vi "Process.vi"(8 "error in":errorcluster, 11 "Qbus in":refnum<class "Qbus.lvclass">) -> (0 "error out":errorcluster)   [LabVIEW 2021, in "TemplateProcess.lvlib"]
uses:
  TemplateProcess.lvlib
  <vilib>/addons/Qbus/Qbus.lvclass
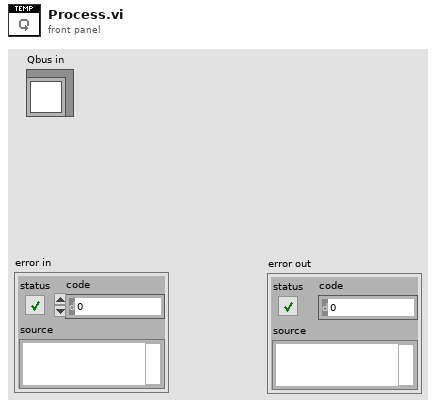
[diagram p1: front panel]
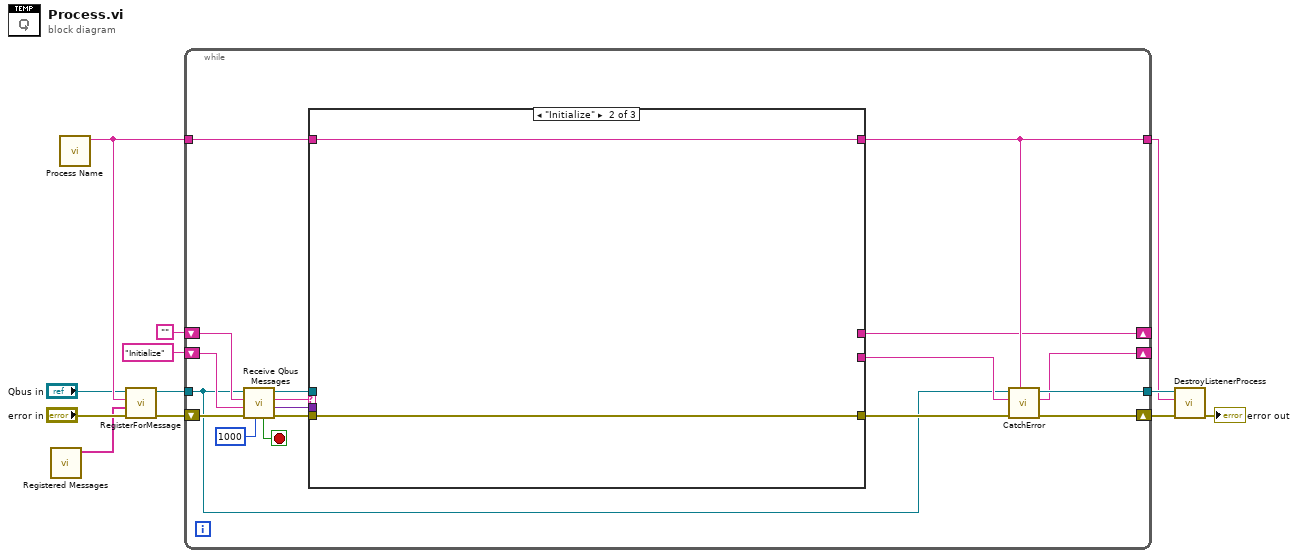
[diagram p0: block diagram]
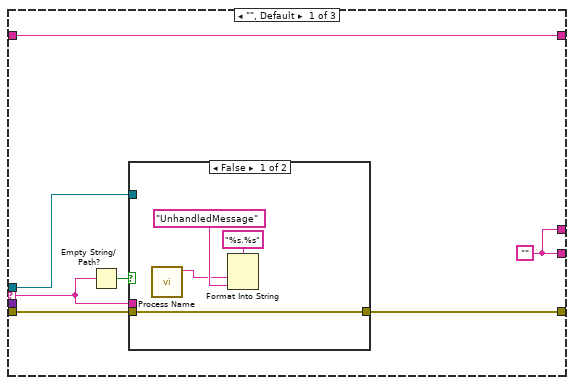
[diagram p2: hidden frame]
diagram:
  n1 = call "Registered Messages.vi"() -> ("registered messages"=w5:string[])  [unwired: 11 in]
  n2 = call "Process Name.vi"() -> ("process name"=w8:string)  [unwired: 11 in]
  n3 = call <vilib>:"RegisterForMessage.vi"("error in (no error)"="error in", "message names"=w5, "process name"=w8, "Qbus in"="Qbus in") -> ("error in (no error)"=w11:errorcluster, "Qbus out"=w12:refnum<class "Qbus.lvclass">)  [unwired: 6 in]
  n4 = while {
    shift-right: [w16] -> _
    shift-left: "" -> [w29]
    tunnel: w12 -> [w14]
    tunnel: w8 -> [w13]
    tunnel: [w23] -> w3
    tunnel: [w18] -> w1
    shift-right: [w22] -> _
    shift-left: "Initialize" -> [w25]
    shift-right: [w24] -> w4
    shift-left: w11 -> [w21]
    stop <- w30 stop-if-true
    n5 = call "Receive Qbus Messages.vi"("timeout(ms)"=1000 ("milliseconds to wait"), "error in (no error)"=w21, "priority action"=w25, "default action"=w29, "Qbus in"=w14) -> ("error out"=w28:errorcluster, "message value"=w26:variant, "action"=w20:string, "Qbus out"=w27:refnum<class "Qbus.lvclass">, "exit"=w30:bool)  [unwired: 2 in]
    n6 = case shown="\"Initialize\"" w20 {
      selector: w20 -> [w34 _ _]
      tunnel: w28 -> [w36 w44 w46]
      tunnel: w27 -> [w32 _ _]
      tunnel: [w35 w44 w46] -> w15
      tunnel: w26 -> [_ _ _]
      tunnel: [w37 w43 w45] -> w18
      tunnel: w13 -> [w37 w43 w45]
      tunnel: [w31 _ _] -> w17
      tunnel: [w31 _ _] -> w16
      frame "", Default {
        w31 = ""
        n7 = Empty String/Path?(string/path=w34) -> (empty?=w33:bool)
        n8 = case shown="False" w33 {
          tunnel: [w38 w42] -> w35
          tunnel: w36 -> [w38 w42]
          tunnel: w34 -> [_ _]
          tunnel: w32 -> [_ _]
          frame False {
            n9 = call "Process Name.vi"() -> ("process name"=w39:string)  [unwired: 11 in]
            n10 = Format Into String(format string="%s.%s", w39, "UnhandledMessage" ("ProcessName")) -> ()  [unwired: 2 in, 2 out]
          }
          frame True {
          }
        }
      }
      frame "Initialize" {
      }
      frame "Exit" {
      }
    }
    n11 = call <vilib>:"CatchError.vi"("source"=w18, "error in (no error)"=w15, "next action in"=w17, "Qbus in"=w14) -> ("error out"=w24:errorcluster, "next action out"=w22:string, "Qbus out"=w23:refnum<class "Qbus.lvclass">)  [unwired: 5 in]
  }
  n12 = call <vilib>:"DestroyListenerProcess.vi"("error in (no error)"=w4, "process name"=w1, "Qbus in"=w3) -> ("error in (no error)"=→"error out":errorcluster)  [unwired: 7 in, 1 out]
